vi "PQconndefaults.vi"(8 "error in (no error)":errorcluster) -> (0 "error out":errorcluster, 3 "PQconninfoOption":u64)   [LabVIEW 2019, in "libpqlv64.lvlib"]
uses:
  libpqlv64.lvlib
  libpq.dll
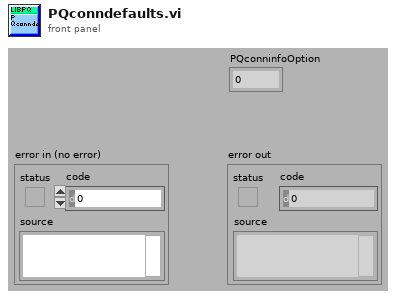
[diagram p1: front panel]
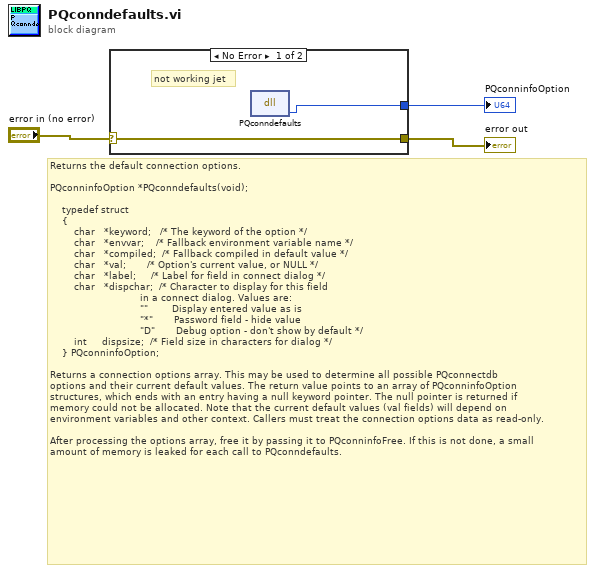
[diagram p0: block diagram]
diagram:
  # "Returns the default connection options.\n\nPQconninfoOption *PQconndefaults(void);\n\n    typedef struct\n    {\n        char   *keyword;   /* The keyword of the option */\n        char   *envvar;    /* Fallback environment variable name */\n        char   *compiled;  /* Fallback compiled in default value */\n        char   *val;       /* Option's current value, or NULL */\n        char   *label;     /* Label for field in connect dialog */\n        char   *dispchar;  /* Character to display for this field\n                              in a connect dialog. Values are:\n                              \"\"        Display entered value as is\n                              \"*\"       Password field - hide value\n                              \"D\"       Debug option - don't show by default */\n        int     dispsize;  /* Field size in characters for dialog */\n    } PQconninfoOption;\n\nReturns a connection options array. This may be used to determine all possible PQconnectdb \noptions and their current default values. The return value points to an array of PQconninfoOption\nstructures, which ends with an entry having a null keyword pointer. The null pointer is returned if \nmemory could not be allocated. Note that the current default values (val fields) will depend on \nenvironment variables and other context. Callers must treat the connection options data as read-only.\n\nAfter processing the options array, free it by passing it to PQconninfoFree. If this is not done, a small \namount of memory is leaked for each call to PQconndefaults."
  n1 = case shown="No Error" "error in (no error)" {
    selector: "error in (no error)" -> [w5 w6]
    tunnel: [w5 w6] -> w2
    tunnel: [w4 _] -> w1
    frame No Error {
      # "not working jet"
      n2 = dll-call lib="libpq.*" fn="PQconndefaults"() -> ("return type"=w4:u64)  [unwired: 3 in, 2 out]
    }
    frame Error {
    }
  }
  "PQconninfoOption" <- w1
  "error out" <- w2
